vi "global_configuration_options.vi"() -> ()   [LabVIEW 2015]
panel:
  in  "Config File Path":path=path "c:/config.txt" caption="配置文件路径"
  in  "Scan Engine Period (us)":u32=20000 caption="扫描引擎周期（微秒）"
  in  "Data File Logging Interval (s)":dbl=5.0 caption="数据文件记录间隔（秒）"
  in  "Error Log Path":path=path "c:/log/log.txt" caption="错误记录路径"
  in  "Data Log Path":path=path "c:/data" caption="数据文件路径"
  in  "Network Stream Buffer Size":i32=50 caption="网络流缓冲区大小"
  in  "Reboot Log Path":path=path "c:/log/reboots.txt" caption="重启记录路径"
  in  "Error Log Duplicate Interval (ms)":u32=5000 caption="错误记录重复间隔（毫秒）"
  in  "Network Stream Polling Timeout (ms)":i32=500 caption="网络流轮询超时（毫秒）"
  in  "Debugging":bool caption="开启调试模式"
  in  "RT Stream Name":string="UI Stream Reader" caption="RT流名称"
  in  "Monitoring Loop Rate (ms)":u32=1000 caption="监测循环频率（毫秒）"
  in  "UI Stream Name":string="UI Stream Writer" caption="UI流名称"
  in  "Network Stream Connect Timeout (ms)":i32=5000 caption="网络流连接超时（毫秒）"
  # "如果修改了任何默认配置选项，必须在保存本VI之前选择编辑>>当前值设为默认值。"
  # "网络流参数设置"
  # "路径设置"
  # "时间参数设置"
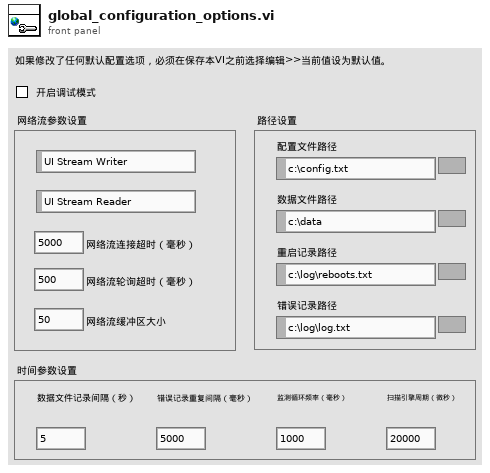
[diagram p1: front panel]
diagram:
